vi "PostScanAction.vi"(0 "Device en entrée":refnum<class "BaseDevice.lvclass"> caption="DNL_LabVIEW Object in", 5 "AcqComp":bool, 7 "ScanDev":bool, 11 "error in (no error)":errorcluster caption="entrée d'erreur (pas d'erreur)") -> (4 "Device en sortie":refnum<class "BaseDevice.lvclass"> caption="DNL_LabVIEW Object out", 6 "PostScanString":string, 15 "error out":errorcluster caption="sortie d'erreur")   [LabVIEW 2019, in "BaseDevice.lvclass"]
uses:
  BaseDevice.lvclass
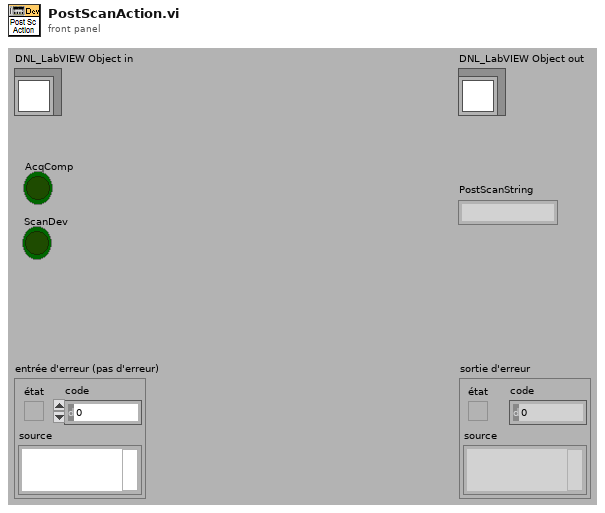
[diagram p1: front panel]
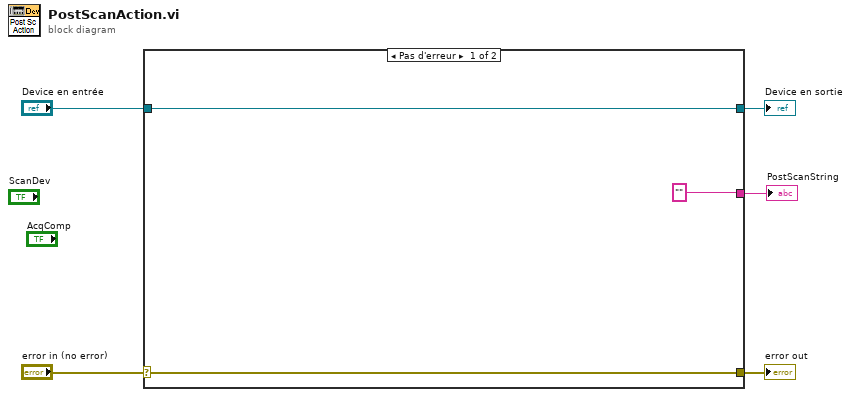
[diagram p0: block diagram]
diagram:
  n1 = case shown="Pas d'erreur" "error in (no error)" {
    selector: "error in (no error)" -> [w8 w10]
    tunnel: [w8 w10] -> w4
    tunnel: [w7 w9] -> w2
    tunnel: "Device en entrée" -> [w7 w9]
    tunnel: ["" _] -> w1
    frame No Error {
    }
    frame Error {
    }
  }
  "error out" <- w4
  "Device en sortie" <- w2
  "PostScanString" <- w1
